vi "clean-change-cursor-kin-event.vi"(1 "cluster in":T1={"Kinetics"=[], "Spectrum"=[], "Experiments groups"=[], "GRAPH EXPERIMENTAL DATA"=[], "error out"={"status"=FALSE, "code"=0, "source"=""}, "group"=0, "exp selected"=0, "# exp"=0, "kinetics plot names"=[], "spectra plot names"=[], "FromToWave"={"FromWave"=0.0, "ToWave"=0.0}, "Laser shutter task"="", "Accelerator task"="", "Motor task"="", "GRAPH EXPERIMENTAL DATA ref"=refnum, "timedelays"=[0.0, 0.0, 0.0, 0.0, 0.0, 0.0, 0.0, 0.06019061100911815, 0.0521779104562645, 0.045231877429679615, 0.03921051490799832, 0.033990728811568754, 0.029465811603150715, 0.025543260876973825, 0.02214288834180205, 0.01919518054014414, 0.016639877791965713, 0.014424742312398925, 0.012504490320209958, 0.010839866306230088, 0.009396840537117498, 0.008145913389103785, 0.00706151229029317, 0.006121468943269439, 0.005306566140927374, 0.004600144911132549, 0.003987763959109073, 0.0034569044455719407, 0.00299671406541447, 0.0025977851951783253, 0.0022519625739982996, 0.00195217658646366, 0.0016922987392150965, 0.0014670163768006634, 0.0012717240756200802, 0.0011024294957352762, 0.0009556717658856477, 0.0008284507332614981, 0.0007181656316962257, 0.0006225619144775864, 0.0005396851648867825, 0.00046784114226338394, 0.0004055611468220084, 0.0003515719951773376, 0.00030476999279031153, 0.00026419837125694315, 0.00022902772919263772, 0.0001985390768670671, 0.0001721091379728629, 0.00014919760805372974, 0.00012933610911736794], "wavelengths"=[0.0, 0.0, 0.0, 0.0, 0.0, 0.0, 0.0, 0.06019061100911815, 0.0521779104562645, 0.045231877429679615, 0.03921051490799832, 0.033990728811568754, 0.029465811603150715, 0.025543260876973825, 0.02214288834180205, 0.01919518054014414, 0.016639877791965713, 0.014424742312398925, 0.012504490320209958, 0.010839866306230088, 0.009396840537117498, 0.008145913389103785, 0.00706151229029317, 0.006121468943269439, 0.005306566140927374, 0.004600144911132549, 0.003987763959109073, 0.0034569044455719407, 0.00299671406541447, 0.0025977851951783253, 0.0022519625739982996, 0.00195217658646366, 0.0016922987392150965, 0.0014670163768006634, 0.0012717240756200802, 0.0011024294957352762, 0.0009556717658856477, 0.0008284507332614981, 0.0007181656316962257, 0.0006225619144775864, 0.0005396851648867825, 0.00046784114226338394, 0.0004055611468220084, 0.0003515719951773376, 0.00030476999279031153, 0.00026419837125694315, 0.00022902772919263772, 0.0001985390768670671, 0.0001721091379728629, 0.00014919760805372974, 0.00012933610911736794], "Experiment"=refnum, "Commentaires exp"=refnum, "FromToDelay"={"FromDelay"=0.0, "ToDelay"=0.0}}, 2 "Kinetics graph":refnum<vi>) -> (0 "cluster out":T1={"Kinetics"=[], "Spectrum"=[], "Experiments groups"=[], "GRAPH EXPERIMENTAL DATA"=[], "error out"={"status"=FALSE, "code"=0, "source"=""}, "group"=0, "exp selected"=0, "# exp"=0, "kinetics plot names"=[], "spectra plot names"=[], "FromToWave"={"FromWave"=0.0, "ToWave"=0.0}, "Laser shutter task"="", "Accelerator task"="", "Motor task"="", "GRAPH EXPERIMENTAL DATA ref"=refnum, "timedelays"=[0.0, 0.0, 0.0, 0.0, 0.0, 0.0, 0.0, 0.06019061100911815, 0.0521779104562645, 0.045231877429679615, 0.03921051490799832, 0.033990728811568754, 0.029465811603150715, 0.025543260876973825, 0.02214288834180205, 0.01919518054014414, 0.016639877791965713, 0.014424742312398925, 0.012504490320209958, 0.010839866306230088, 0.009396840537117498, 0.008145913389103785, 0.00706151229029317, 0.006121468943269439, 0.005306566140927374, 0.004600144911132549, 0.003987763959109073, 0.0034569044455719407, 0.00299671406541447, 0.0025977851951783253, 0.0022519625739982996, 0.00195217658646366, 0.0016922987392150965, 0.0014670163768006634, 0.0012717240756200802, 0.0011024294957352762, 0.0009556717658856477, 0.0008284507332614981, 0.0007181656316962257, 0.0006225619144775864, 0.0005396851648867825, 0.00046784114226338394, 0.0004055611468220084, 0.0003515719951773376, 0.00030476999279031153, 0.00026419837125694315, 0.00022902772919263772, 0.0001985390768670671, 0.0001721091379728629, 0.00014919760805372974, 0.00012933610911736794], "wavelengths"=[0.0, 0.0, 0.0, 0.0, 0.0, 0.0, 0.0, 0.06019061100911815, 0.0521779104562645, 0.045231877429679615, 0.03921051490799832, 0.033990728811568754, 0.029465811603150715, 0.025543260876973825, 0.02214288834180205, 0.01919518054014414, 0.016639877791965713, 0.014424742312398925, 0.012504490320209958, 0.010839866306230088, 0.009396840537117498, 0.008145913389103785, 0.00706151229029317, 0.006121468943269439, 0.005306566140927374, 0.004600144911132549, 0.003987763959109073, 0.0034569044455719407, 0.00299671406541447, 0.0025977851951783253, 0.0022519625739982996, 0.00195217658646366, 0.0016922987392150965, 0.0014670163768006634, 0.0012717240756200802, 0.0011024294957352762, 0.0009556717658856477, 0.0008284507332614981, 0.0007181656316962257, 0.0006225619144775864, 0.0005396851648867825, 0.00046784114226338394, 0.0004055611468220084, 0.0003515719951773376, 0.00030476999279031153, 0.00026419837125694315, 0.00022902772919263772, 0.0001985390768670671, 0.0001721091379728629, 0.00014919760805372974, 0.00012933610911736794], "Experiment"=refnum, "Commentaires exp"=refnum, "FromToDelay"={"FromDelay"=0.0, "ToDelay"=0.0}})   [LabVIEW 2015]
uses:
  controls/control-cluster.ctl
  Classes/Experiments_group.lvclass
  Classes/Experiment.lvclass
types:
  T1 = typedef "control-cluster.ctl" = cluster{"Kinetics":cluster{"timedelay":dbl[], dbl[]}[], "Spectrum":cluster{"Unités abscisse":dbl[], dbl[]}[], "Experiments groups":refnum<class "Experiments_group.lvclass">[], "GRAPH EXPERIMENTAL DATA":dbl[][], "error out":errorcluster, "group":i32, "exp selected":i32, "# exp":i32, "kinetics plot names":string[], "spectra plot names":string[], "FromToWave":cluster{"FromWave":dbl, "ToWave":dbl}, "Laser shutter task":refnum<k21>, "Accelerator task":refnum<k21>, "Motor task":refnum<k21>, "GRAPH EXPERIMENTAL DATA ref":refnum<vi>, "timedelays":dbl[], "wavelengths":dbl[], "Experiment":refnum<vi>, "Commentaires exp":refnum<vi>, "FromToDelay":cluster{"FromDelay":dbl, "ToDelay":dbl}}
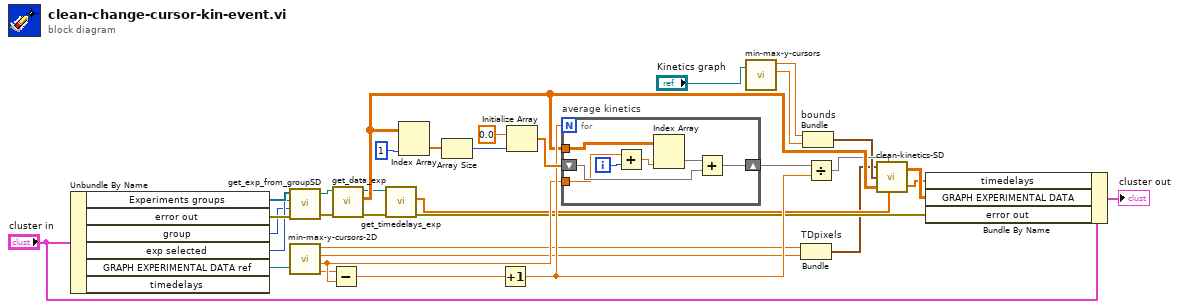
[diagram p0: block diagram]
diagram:
  n1 = Unbundle By Name("cluster in") -> ("Experiments groups"=w33:refnum<class "Experiments_group.lvclass">[], "error out"=w32:errorcluster, "group"=w29:i32, "exp selected"=w30:i32, "GRAPH EXPERIMENTAL DATA ref"=w14:refnum<vi>)  [unwired: 1 out]
  n2 = call "get_exp_from_groupSD.vi"("error in (no error)"=w32, "group"=w29, "exp selected"=w30, "Experiments groups"=w33) -> ("error out"=w16:errorcluster, "Experiment out"=w17:refnum<class "Experiment.lvclass">)  [unwired: 1 out]
  n3 = call "min-max-y-cursors-2D.vi"("GRAPH EXPERIMENTAL DATA ref"=w14) -> ("minY"=w4:dbl, "maxY"=w3:dbl, "minX"=w13:dbl, "maxX"=w12:dbl)  [unwired: 1 in]
  n4 = Subtract(x=w12, y=w13) -> (x-y=w20:dbl)
  n5 = call-dynamic "get_data_exp.vi"("error in (no error)"=w16, "Experiment.lvclass in"=w17) -> ("error out"=w9:errorcluster, "Data"=w18:dbl[][], "Experiment.lvclass out"=w10:refnum<class "Experiment.lvclass">)  [unwired: 7 in]
  n6 = call-dynamic "get_timedelays_exp.vi"("error in (no error)"=w9, "Experiment.lvclass in"=w10) -> ("error out"=w8:errorcluster, "timedelays"=w7:dbl[])  [unwired: 7 in, 1 out]
  n7 = Index Array(array=w18, index (col)=1 ("disabled index (col)")) -> (element=w22:dbl[])  [unwired: 1 in]
  n8 = Array Size(array=w22) -> (size(s)=w24:i32)
  n9 = Increment(x=w20) -> (x+1=w19:dbl)
  n10 = Initialize Array(0.0 ("element"), w24) -> (w21:dbl[])
  n11 = for "average kinetics" {
    N: w19 -> [_]
    tunnel: w18 -> [w41]
    shift-right: [w36] -> w25
    shift-left: w21 -> [w37]
    tunnel: w13 -> [w35]
    i -> [w40]
    n12 = Add(x=w35, y=w40) -> (x+y=w39:dbl)
    n13 = Index Array(array=w41, index (col)=w39) -> (element=w38:dbl[])  [unwired: 1 in]
    n14 = Add(x=w38, y=w37) -> (x+y=w36:dbl[])
  }
  n15 = call "min-max-y-cursors.vi"("XYGraph in"="Kinetics graph") -> ("minY"=w6:dbl, "maxY"=w5:dbl)  [unwired: 1 in, 2 out]
  n16 = Bundle "TDpixels"("minY"=w4, "maxY"=w3) -> (w1:cluster{"minY":dbl, "maxY":dbl})  [unwired: 1 in]
  n17 = Bundle "bounds"("minY"=w6, "maxY"=w5) -> (w2:cluster{"minY":dbl, "maxY":dbl})  [unwired: 1 in]
  n18 = Divide(x=w25, y=w19) -> (x/y=w15:dbl[])
  n19 = call "clean-kinetics-SD.vi"("TDpixels"=w1, "kinetics"=w15, "bounds"=w2, "Data"=w18, "timedelays"=w7) -> ("Data out"=w31:dbl[][], "timedelays out"=w11:dbl[])
  n20 = Bundle By Name(cluster="cluster in", "timedelays"=w11, "GRAPH EXPERIMENTAL DATA"=w31, "error out"=w8) -> (→"cluster out":T1)
